vi "Rectangulo_Init.vi"(8 "Error In":errorcluster, 11 "object in":refnum<class "Rectangulo.lvclass">) -> (0 "Error Out":errorcluster, 3 "object out":refnum<class "Rectangulo.lvclass">)   [LabVIEW 2024, in "Rectangulo.lvclass"]
uses:
  Rectangulo.lvclass
  Rectangulo.lvclass/Rectangulo.ctl
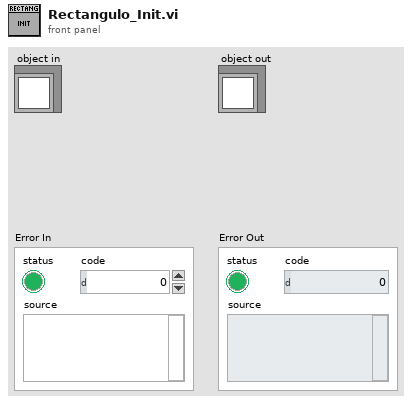
[diagram p1: front panel]
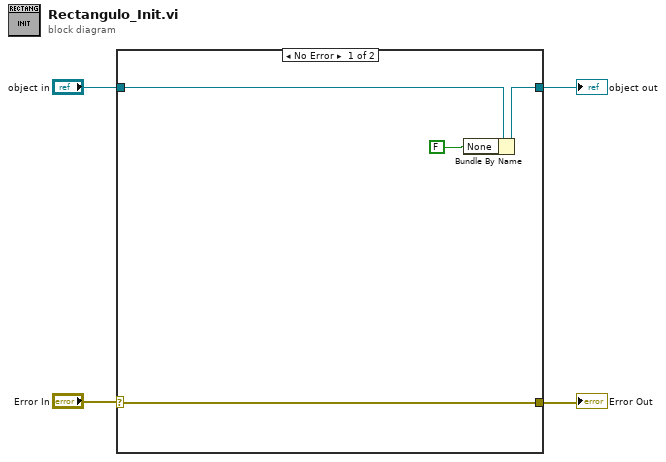
[diagram p0: block diagram]
diagram:
  n1 = case shown="No Error" "Error In" {
    selector: "Error In" -> [w5 w9]
    tunnel: "object in" -> [w8 w10]
    tunnel: [w7 w10] -> w3
    tunnel: [w5 w9] -> w1
    frame No Error {
      n2 = Bundle By Name(cluster=w8, "None"=FALSE) -> (w7:refnum<class "Rectangulo.lvclass">)
    }
    frame Error {
    }
  }
  "object out" <- w3
  "Error Out" <- w1
